vi "전자레인지.vi"() -> ()   [LabVIEW 2020]
panel:
  in  "조리시작":bool
  in  "문열림":bool
  in  "정지":bool
  in  "1분":bool
  out "시간":string
  in  "30초":bool
  in  "10초":bool
  out "전자레인지 Light":bool
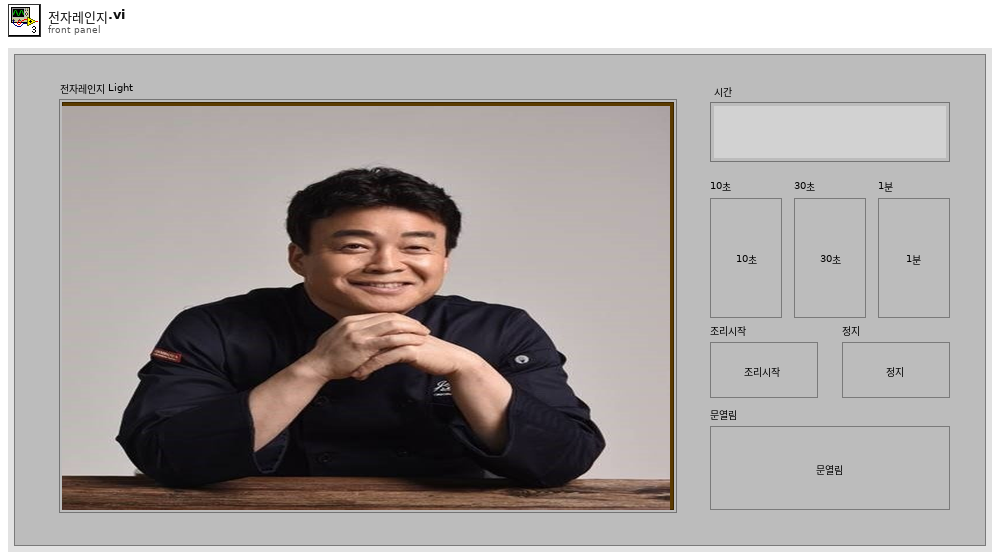
[diagram p1: front panel]
types:
  T1 = cluster{"30초":bool, "1분":bool, "정지":bool, "문열림":bool, "시간":string, "전자레인지 Light":bool}
  T2 = typedef "컨트롤 2.ctl" = enum16{"초기화", "디스플레이 업데이트", "10초", "30초", "1분", "조리시작", "문열림", "정지"}
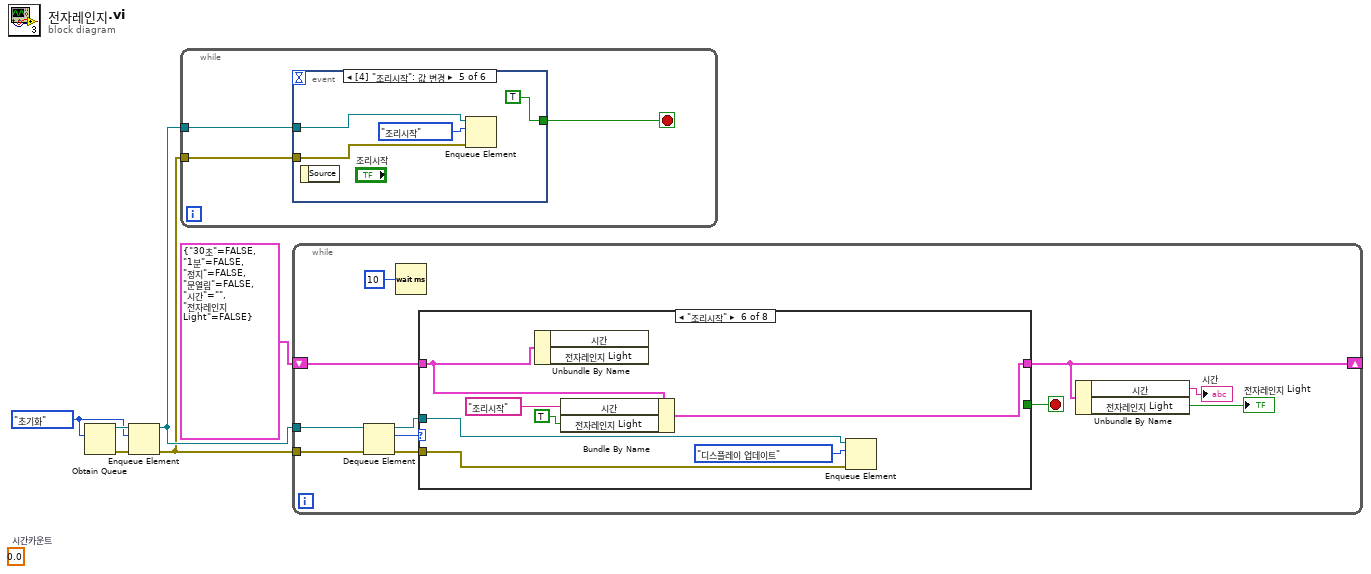
[diagram p0: block diagram]
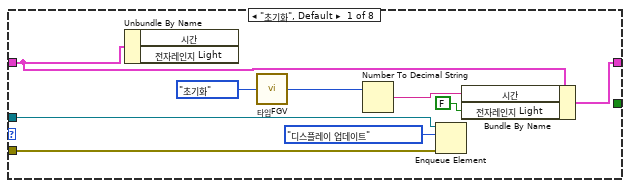
[diagram p2: hidden frame]
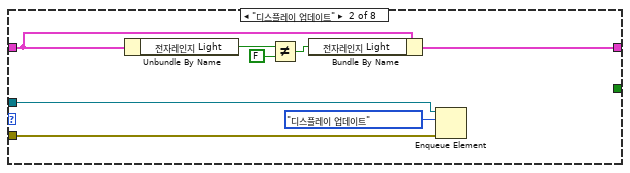
[diagram p3: hidden frame]
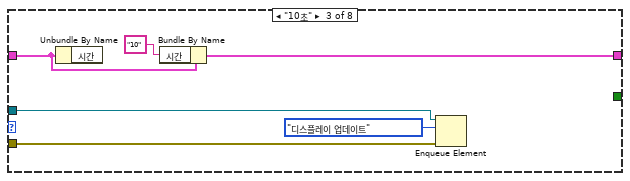
[diagram p4: hidden frame]
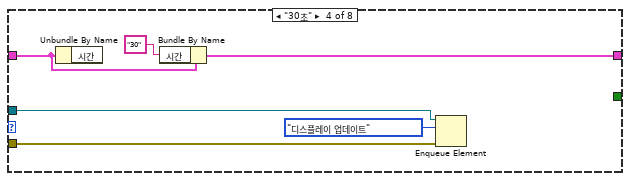
[diagram p5: hidden frame]
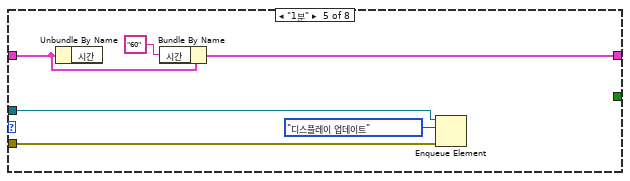
[diagram p6: hidden frame]
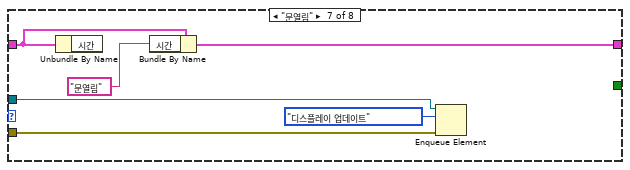
[diagram p7: hidden frame]
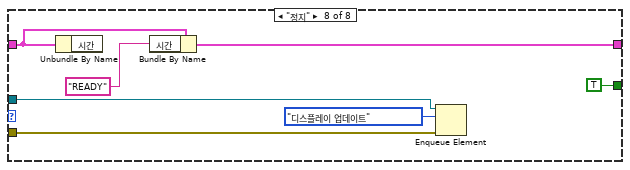
[diagram p8: hidden frame]
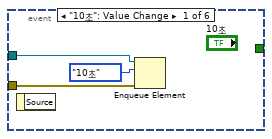
[diagram p9: hidden frame]
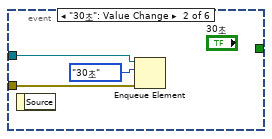
[diagram p10: hidden frame]
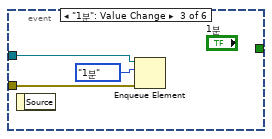
[diagram p11: hidden frame]
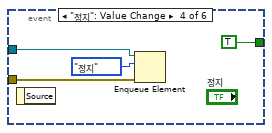
[diagram p12: hidden frame]
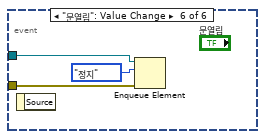
[diagram p13: hidden frame]
diagram:
  (unwired) 0.0  # 시간카운트
  w4 = 컨트롤_2."초기화"
  n1 = Obtain Queue(element data type=w4) -> (queue out=w6:refnum<queue>, error out=w5:errorcluster)  [unwired: 4 in, 1 out]
  n2 = Enqueue Element(queue=w6, element=w4, error in (no error)=w5) -> (queue out=w3:refnum<queue>, error out=w2:errorcluster)  [unwired: 1 in, 1 out]
  n3 = while {
    tunnel: w3 -> [w9]
    tunnel: w2 -> [w8]
    stop <- w7 stop-if-true
    n4 = event shown="[4] \"조리시작\": 값 변경" {
      selector: _ -> [_ _ _ _ _ _]
      dyn-events: _ -> [_ _ _ _ _ _]
      timeout: _ -> [_ _ _ _ _ _]
      tunnel: w9 -> [w12 w15 w18 w22 w26 w29]
      tunnel: w8 -> [w11 w14 w17 w21 w25 w28]
      tunnel: [_ _ _ TRUE TRUE _] -> w7
      event "10초": Value Change {
        n5 = event-data() -> ()  [unwired: 1 in, 1 out]
        n6 = Enqueue Element(queue=w12, element=컨트롤_2."10초", error in (no error)=w11) -> ()  [unwired: 1 in, 3 out]
      }
      event "30초": Value Change {
        n7 = event-data() -> ()  [unwired: 1 in, 1 out]
        n8 = Enqueue Element(queue=w15, element=컨트롤_2."30초", error in (no error)=w14) -> ()  [unwired: 1 in, 3 out]
      }
      event "1분": Value Change {
        n9 = event-data() -> ()  [unwired: 1 in, 1 out]
        n10 = Enqueue Element(queue=w18, element=컨트롤_2."1분", error in (no error)=w17) -> ()  [unwired: 1 in, 3 out]
      }
      event "정지": Value Change {
        n11 = event-data() -> ()  [unwired: 1 in, 1 out]
        n12 = Enqueue Element(queue=w22, element=컨트롤_2."정지", error in (no error)=w21) -> ()  [unwired: 1 in, 3 out]
      }
      event "조리시작": Value Change {
        n13 = event-data() -> ()  [unwired: 1 in, 1 out]
        n14 = Enqueue Element(queue=w26, element=컨트롤_2."조리시작", error in (no error)=w25) -> ()  [unwired: 1 in, 3 out]
      }
      event "문열림": Value Change {
        n15 = event-data() -> ()  [unwired: 1 in, 1 out]
        n16 = Enqueue Element(queue=w29, element=컨트롤_2."정지", error in (no error)=w28) -> ()  [unwired: 1 in, 3 out]
      }
    }
  }
  n17 = while {
    tunnel: w3 -> [w39]
    tunnel: w2 -> [w38]
    shift-right: [w32] -> _
    shift-left: T1 {"30초"=FALSE, "1분"=FALSE, "정지"=FALSE, "문열림"=FALSE, "시간"="", "전자레인지 Light"=FALSE} -> [w40]
    stop <- w31 stop-if-true
    n18 = Dequeue Element(queue=w39, error in (no error)=w38) -> (queue out=w37:refnum<queue>, element=w35:T2, error out=w36:errorcluster)  [unwired: 1 in, 1 out]
    n19 = Wait (ms)(milliseconds to wait=u32 10 ("대기 시간 (ms)")) -> ()  [unwired: 1 out]
    n20 = case shown="\"조리시작\"" w35 {
      tunnel: w40 -> [w46 w54 w60 w65 w71 w79 w85 w91]
      tunnel: w37 -> [w49 w56 w58 w67 w73 w81 w87 w93]
      tunnel: w36 -> [w48 w55 w59 w66 w72 w80 w86 w92]
      tunnel: [w45 w53 w61 w64 w70 w78 w84 w90] -> w32
      tunnel: [_ _ _ _ _ _ _ TRUE] -> w31
      frame "초기화", Default {
        n21 = Unbundle By Name(w46) -> ()  [unwired: 2 out]
        n22 = call "타임FGV.vi"("열거형"=enum16{"초기화", "카운트", "정지"}."초기화") -> ("카운트"=w42:u32)
        n23 = Number To Decimal String(number=w42) -> (decimal integer string=w41:string)  [unwired: 1 in]
        n24 = Enqueue Element(queue=w49, element=컨트롤_2."디스플레이 업데이트", error in (no error)=w48) -> ()  [unwired: 1 in, 3 out]
        n25 = Bundle By Name(cluster=w46, "시간"=w41, "전자레인지 Light"=FALSE) -> (w45:T1)
      }
      frame "디스플레이 업데이트" {
        n26 = Unbundle By Name(w54) -> ("전자레인지 Light"=w52:bool)
        n27 = Not Equal?(x=w52, y=FALSE) -> (x != y?=w51:bool)
        n28 = Bundle By Name(cluster=w54, "전자레인지 Light"=w51) -> (w53:T1)
        n29 = Enqueue Element(queue=w56, element=컨트롤_2."디스플레이 업데이트", error in (no error)=w55) -> ()  [unwired: 1 in, 3 out]
      }
      frame "10초" {
        n30 = Unbundle By Name(w60) -> ()  [unwired: 1 out]
        n31 = Bundle By Name(cluster=w60, "시간"="10") -> (w61:T1)
        n32 = Enqueue Element(queue=w58, element=컨트롤_2."디스플레이 업데이트", error in (no error)=w59) -> ()  [unwired: 1 in, 3 out]
      }
      frame "30초" {
        n33 = Unbundle By Name(w65) -> ()  [unwired: 1 out]
        n34 = Bundle By Name(cluster=w65, "시간"="30") -> (w64:T1)
        n35 = Enqueue Element(queue=w67, element=컨트롤_2."디스플레이 업데이트", error in (no error)=w66) -> ()  [unwired: 1 in, 3 out]
      }
      frame "1분" {
        n36 = Unbundle By Name(w71) -> ()  [unwired: 1 out]
        n37 = Bundle By Name(cluster=w71, "시간"="60") -> (w70:T1)
        n38 = Enqueue Element(queue=w73, element=컨트롤_2."디스플레이 업데이트", error in (no error)=w72) -> ()  [unwired: 1 in, 3 out]
      }
      frame "조리시작" {
        n39 = Unbundle By Name(w79) -> ()  [unwired: 2 out]
        n40 = Bundle By Name(cluster=w79, "시간"="조리시작", "전자레인지 Light"=TRUE) -> (w78:T1)
        n41 = Enqueue Element(queue=w81, element=컨트롤_2."디스플레이 업데이트", error in (no error)=w80) -> ()  [unwired: 1 in, 3 out]
      }
      frame "문열림" {
        n42 = Unbundle By Name(w85) -> ()  [unwired: 1 out]
        n43 = Bundle By Name(cluster=w85, "시간"="문열림") -> (w84:T1)
        n44 = Enqueue Element(queue=w87, element=컨트롤_2."디스플레이 업데이트", error in (no error)=w86) -> ()  [unwired: 1 in, 3 out]
      }
      frame "정지" {
        n45 = Unbundle By Name(w91) -> ()  [unwired: 1 out]
        n46 = Bundle By Name(cluster=w91, "시간"="READY") -> (w90:T1)
        n47 = Enqueue Element(queue=w93, element=컨트롤_2."디스플레이 업데이트", error in (no error)=w92) -> ()  [unwired: 1 in, 3 out]
      }
    }
    n48 = Unbundle By Name(w32) -> ("시간"=→"시간":string, "전자레인지 Light"=→"전자레인지 Light":bool)
  }
